vi "Create Events.vi"(0 "Display State In":T2, 9 "Container State":T3, 11 "error in (no error)":errorcluster) -> (4 "Display State Out":T2, 8 "Events":T1, 15 "error out":errorcluster)   [LabVIEW 2020, in "Input Criterion.xctl"]
uses:
  Input Criterion.xctl
  <vilib>/_xctls/Container State.ctl
  State.vi
  Events.ctl
  Event Type.ctl
  Operator.vi
  Digital Input VIs/Tosca-Input Criterion.ctl
  epl-vi-lib/Utility VIs/Type Defs/Logic State.ctl
  Event Data.ctl
  Criterion.vi
  <vilib>/_xctls/XControlSupport.lvlib
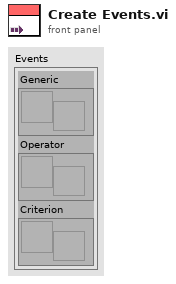
[diagram p1: front panel]
types:
  T1 = typedef "Input Criterion.xctl/Events.ctl" = cluster{"Generic":refnum<user-event>, "Operator":refnum<user-event>, "Criterion":refnum<user-event>}
  T2 = typedef "Input Criterion.xctl/State.vi" = cluster{"DI":string[], "Flags":string[], "show op":bool, "flag start":i16, "Events":T1}
  T3 = typedef "XControlSupport.lvlib/Container State.ctl" = cluster{"Indicator?":bool, "Run Mode?":bool, " Refnum":refnum<vi>}
  T4 = typedef "Input Criterion.xctl/Criterion.vi" = cluster{"Criterion":T5}
  T5 = typedef "Tosca-Input Criterion.ctl" = cluster{"DigInput":i32, "State":T6, "Time (ms)":i32, "Name":string}
  T6 = typedef "Logic State.ctl" = enum16{"Low", "High", "Rising", "Falling"}
  T7 = typedef "Input Criterion.xctl/Operator.vi" = cluster{"Value":i16}
  T8 = typedef "Input Criterion.xctl/Event Data.ctl" = cluster{"Type":T9, "Data":variant}
  T9 = typedef "Input Criterion.xctl/Event Type.ctl" = enum16{"None", "Selection", "Edit", "Insert", "Delete", "Up", "Down"}
  T10 = cluster{"Event Data":refnum<user-event>, "Event Data":refnum<user-event>, "Event Data":refnum<user-event>}
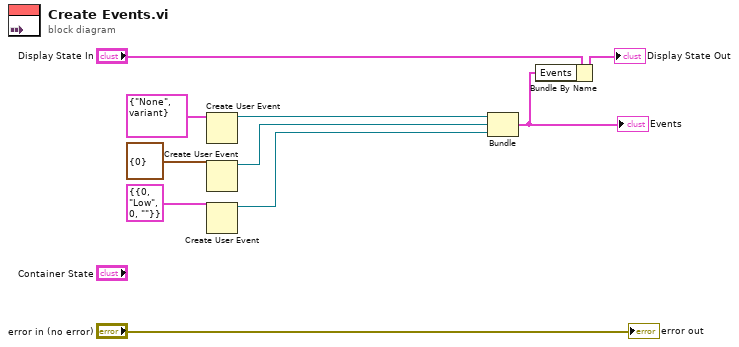
[diagram p0: block diagram]
diagram:
  n1 = Create User Event(user event datatype=T8 {"Type"=enum."None", "Data"=variant} ("Event Data")) -> (user event=w6:refnum<user-event>)  [unwired: 1 in, 1 out]
  n2 = Create User Event(user event datatype=T7 {"Value"=0} ("Event Data")) -> (user event=w4:refnum<user-event>)  [unwired: 1 in, 1 out]
  n3 = Create User Event(user event datatype=T4 {"Criterion"={"DigInput"=0, "State"=enum."Low", "Time (ms)"=0, "Name"=""}} ("Event Data")) -> (user event=w1:refnum<user-event>)  [unwired: 1 in, 1 out]
  n4 = Bundle("Event Data"=w6, "Event Data"=w4, "Event Data"=w1) -> (w3:T10)  [unwired: 1 in]
  "Events" <- w3
  n5 = Bundle By Name(cluster="Display State In", "Events"=w3) -> (→"Display State Out":T2)
  "error out" <- "error in (no error)"
